vi "guitarscales.vi"(10 "Project Detail 2":T1, 11 "Notes in Scale in":bool[](array[boolean])) -> ()   [LabVIEW 2019]
uses:
  Project Parameters.ctl
panel:
  out "E":bool[](array[boolean])
  out "A":bool[](array[boolean])
  out "D":bool[](array[boolean])
  out "G":bool[](array[boolean])
  out "B":bool[](array[boolean])
  out "e":bool[](array[boolean])
  # "e\n\nB\n\nG\n\nD\n\nA\n\nE"
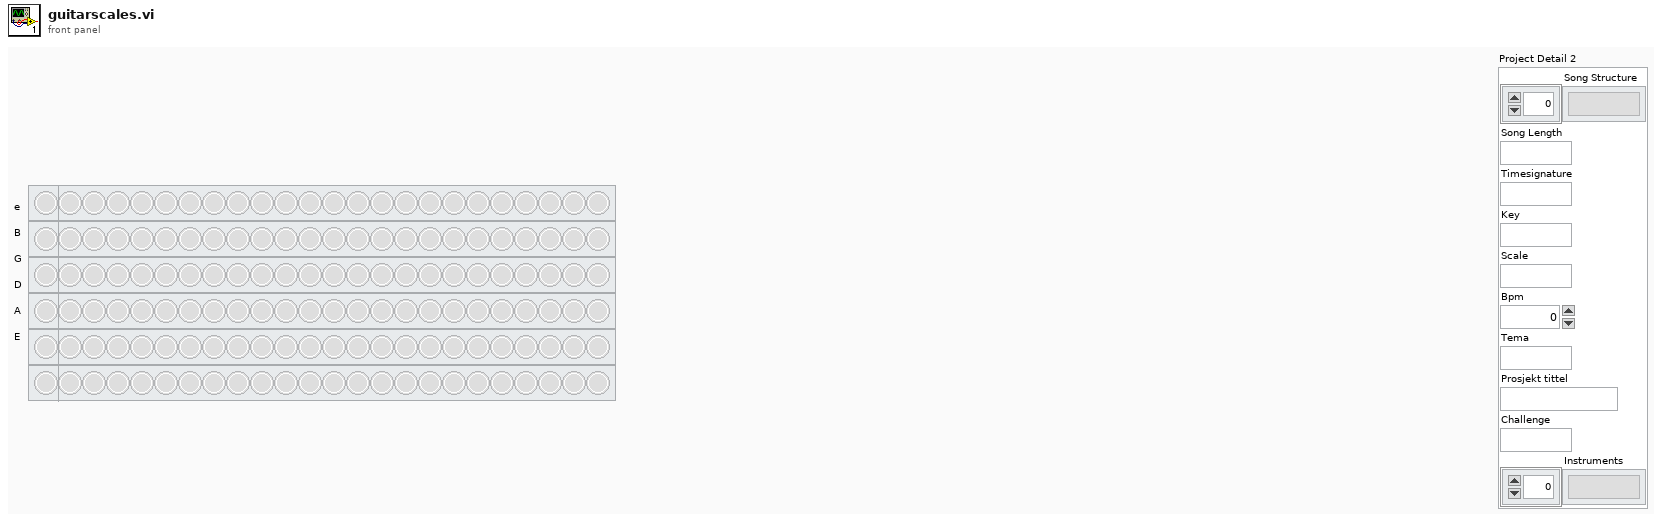
[diagram p1: front panel]
types:
  T1 = typedef "Project Parameters.ctl" = cluster{"Song Structure":string[], "Song Length":string, "Timesignature":string, "Key":string, "Scale":string, "Bpm":i32, "Tema":string, "Prosjekt tittel":string, "Challenge":string, "Instruments":string[]}
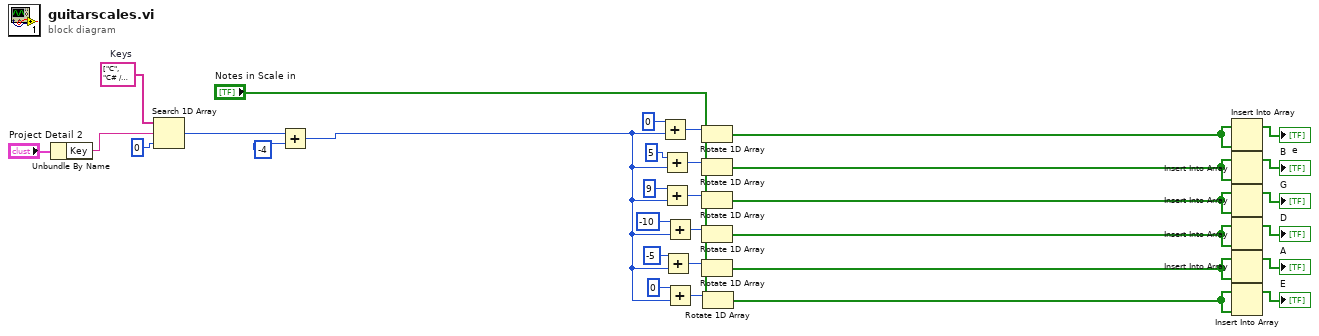
[diagram p0: block diagram]
diagram:
  w4 = string[] ["C", "C# / Db", "D", "D# / Eb", "E", "F", "F# / Gb", "G", "G# / Ab", "A", "A# / Bb", "B"]  # Keys
  n1 = Unbundle By Name("Project Detail 2") -> ("Key"=w13:string)
  n2 = Search 1D Array(1D array=w4, element=w13, start index (0)=0) -> (index of element=w3:i32)
  n3 = Add(x=w3, y=-4) -> (x+y=w2:i32)
  n4 = Add(x=0 ("n"), y=w2) -> (x+y=w19:i32)
  n5 = Add(x=5 ("n"), y=w2) -> (x+y=w17:i32)
  n6 = Add(x=9 ("n"), y=w2) -> (x+y=w16:i32)
  n7 = Add(x=-5 ("n"), y=w2) -> (x+y=w15:i32)
  n8 = Add(x=-10 ("n 2"), y=w2) -> (x+y=w14:i32)
  n9 = Add(x=0 ("n"), y=w2) -> (x+y=w18:i32)
  n10 = Rotate 1D Array(1:"Notes in Scale in", 2:w19) -> (0:w21:bool[])
  n11 = Rotate 1D Array(1:"Notes in Scale in", 2:w17) -> (0:w22:bool[])
  n12 = Rotate 1D Array(1:"Notes in Scale in", 2:w16) -> (0:w24:bool[])
  n13 = Rotate 1D Array(1:"Notes in Scale in", 2:w14) -> (0:w25:bool[])
  n14 = Rotate 1D Array(1:"Notes in Scale in", 2:w15) -> (0:w26:bool[])
  n15 = Rotate 1D Array(1:"Notes in Scale in", 2:w18) -> (0:w27:bool[])
  n16 = Insert Into Array(array=w21, new element=w21) -> (→"e":bool[])  [unwired: 1 in]
  n17 = Insert Into Array(array=w22, new element=w22) -> (→"B":bool[])  [unwired: 1 in]
  n18 = Insert Into Array(array=w24, new element=w24) -> (→"G":bool[])  [unwired: 1 in]
  n19 = Insert Into Array(array=w25, new element=w25) -> (→"D":bool[])  [unwired: 1 in]
  n20 = Insert Into Array(array=w26, new element=w26) -> (→"A":bool[])  [unwired: 1 in]
  n21 = Insert Into Array(array=w27, new element=w27) -> (→"E":bool[])  [unwired: 1 in]
